vi "VCS Wait For Target Reached.vi"(8 "error in (no error)":errorcluster, 9 "timeout":u32, 11 "axis in":cluster{"keyHandle":u32, "nodeId":u16}={"keyHandle"=0, "nodeId"=1}) -> (0 "error out":errorcluster, 3 "axis out":cluster{"keyHandle":u32, "nodeId":u16}={"keyHandle"=0, "nodeId"=1})   [LabVIEW 2019]
doc: "<B>VCS_WaitForTargetReached</B> is waiting until the state is changed to target reached or the time is up."
uses:
  Resources/EposCmd.dll
  Resources/EposCmd64.dll
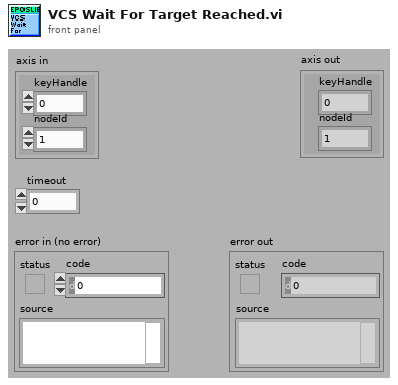
[diagram p1: front panel]
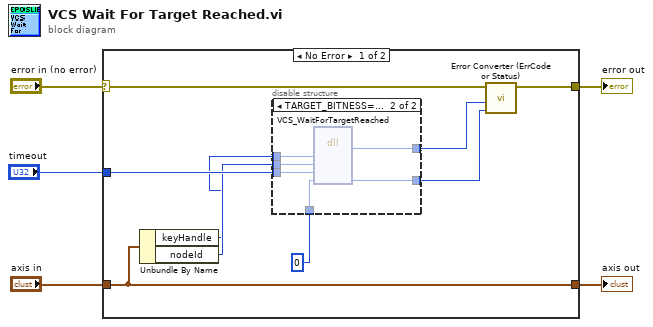
[diagram p0: block diagram]
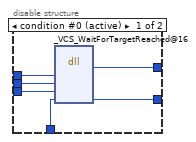
[diagram p2: hidden frame]
diagram:
  n1 = case shown="No Error" "error in (no error)" {
    selector: "error in (no error)" -> [w12 w27]
    tunnel: "axis in" -> [w14 w28]
    tunnel: [w14 w28] -> w4
    tunnel: [w13 w27] -> w3
    tunnel: "timeout" -> [w10 _]
    frame No Error {
      n2 = Unbundle By Name(w14) -> ("keyHandle"=w6:u32, "nodeId"=w9:u16)
      n3 = disable-structure shown="TARGET_BITNESS==64" {
        disable-tunnel: u32 0 ("pErrorCode") -> [w20 w26]
        disable-tunnel: w10 -> [w19 w25]
        disable-tunnel: w9 -> [w18 w24]
        disable-tunnel: [w17 w23] -> w8
        disable-tunnel: [w16 w22] -> w7
        disable-tunnel: w6 -> [w15 w21]
        frame condition #0 (active) {
          n4 = dll-call lib="C:/Projeto em LabVIEW/EPOS-LabVIEW-Instrument-Driver-En/LabVIEW/maxon EPOS/Resources/EposCmd.*" fn="_VCS_WaitForTargetReached@16"("KeyHandle"=w15, "NodeId"=w18, "Timeout"=w19, "pErrorCode"=w20) -> ("Rückgabetyp"=w17:i32, "pErrorCode"=w16:u32)  [unwired: 6 in, 2 out]
        }
        frame condition #1 {
          n5 = dll-call lib="C:/setup/Resources/EposCmd64.*" fn="VCS_WaitForTargetReached" ("EposCmd.dll:_VCS_WaitForTargetReached@16")("KeyHandle"=w21, "NodeId"=w24, "Timeout"=w25, "pErrorCode"=w26) -> ("Rückgabetyp"=w23:i32, "pErrorCode"=w22:u32)  [unwired: 6 in, 2 out]
        }
      }
      n6 = call "Error Converter (ErrCode or Status).vi"("error code"=w7, "return type"=w8, "error in (no error)"=w12) -> ("error out"=w13:errorcluster)  [unwired: 7 in]
    }
    frame Error {
    }
  }
  "error out" <- w3
  "axis out" <- w4
